vi "Transmit Transfer Data.vi"(5 "transfer id":i32, 7 "transfer group id":i32, 8 "error in":errorcluster, 9 "transfer data":u8[](array[numeric]), 11 "RDMA Transceiver in":refnum<class "RDMA Transceiver.lvclass">) -> (0 "error out":errorcluster, 1 "timed out?":bool, 3 "RDMA Transceiver out":refnum<class "RDMA Transceiver.lvclass">)   [LabVIEW 2020, in "RDMA.lvlib" / "RDMA Transceiver.lvclass"]
doc: "Writes transfer data to RDMA buffer"
uses:
  RDMA Transceiver.lvclass
  <vilib>/Utility/error.llb/Clear Errors.vi
  RDMA Transceiver.lvclass/RDMA Transceiver.ctl
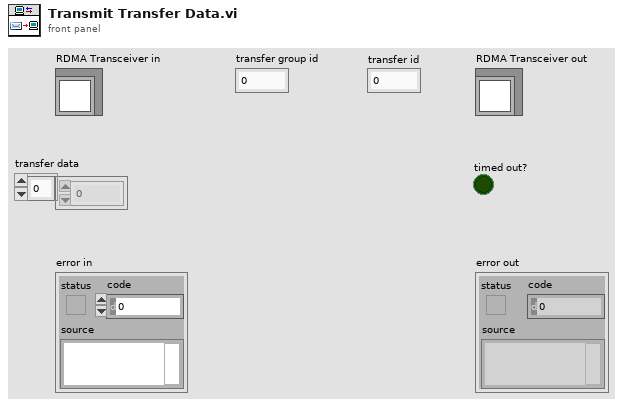
[diagram p1: front panel]
types:
  T1 = typedef "RDMA.lvlib/RDMA Transceiver.lvclass/Transfer Group Parameters.ctl" = cluster{"transfers":T2[]}
  T2 = typedef "RDMA.lvlib/RDMA Transceiver.lvclass/Transfer Parameters.ctl" = cluster{"connected session":refnum<k21>, "listener session":refnum<k21>}
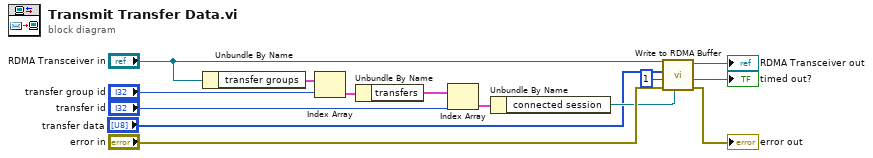
[diagram p0: block diagram]
diagram:
  n1 = Unbundle By Name("RDMA Transceiver in") -> ("transfer groups"=w14:T1[])
  n2 = Index Array(array=w14, index="transfer group id") -> (element=w13:T1)
  n3 = Unbundle By Name(w13) -> ("transfers"=w11:T2[])
  n4 = Index Array(array=w11, index="transfer id") -> (element=w12:T2)
  n5 = Unbundle By Name(w12) -> ("connected session"=w2:refnum<k21>)
  n6 = call "Write to RDMA Buffer.vi"("rdma session"=w2, "error in"="error in", "timeout ms (25000)"=1, "data"="transfer data", "RDMA Transceiver in"="RDMA Transceiver in") -> ("error out"=→"error out":errorcluster, "timed out?"=→"timed out?":bool, "RDMA Transceiver out"=→"RDMA Transceiver out":refnum<class "RDMA Transceiver.lvclass">)  [unwired: 4 in]
